vi "Write Sub Panel.vi"(8 "error in (no error)":errorcluster, 10 "Sub Panel":refnum<vi>, 11 "Window with subpanel in":refnum<class "Window with subpanel.lvclass">) -> (0 "error out":errorcluster, 3 "Window with subpanel out":refnum<class "Window with subpanel.lvclass">)   [LabVIEW 2020, in "Panel Form Tier Controllers.lvlib" / "Window with subpanel.lvclass"]
uses:
  Window with subpanel.lvclass
  Window with subpanel.lvclass/Window with subpanel.ctl
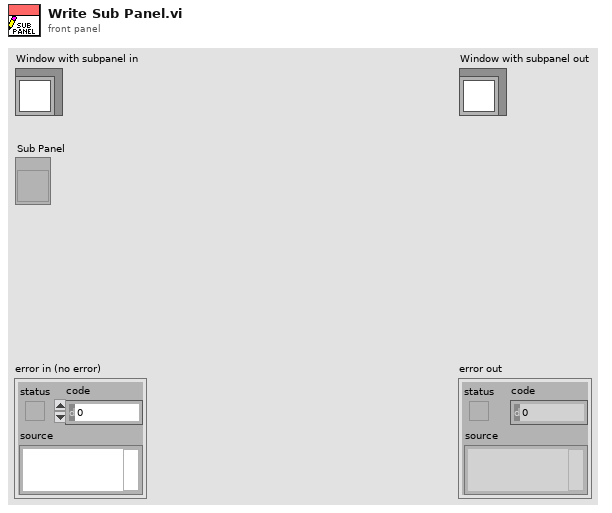
[diagram p1: front panel]
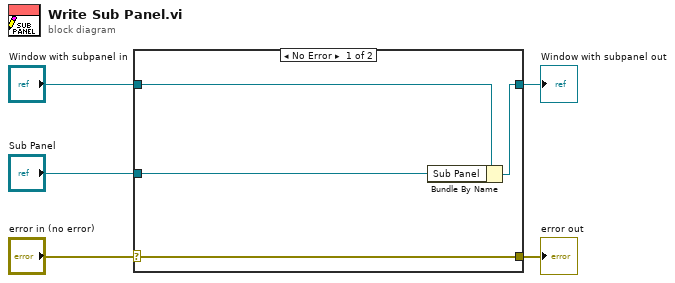
[diagram p0: block diagram]
diagram:
  n1 = case shown="No Error" "error in (no error)" {
    selector: "error in (no error)" -> [w9 w10]
    tunnel: [w9 w10] -> w4
    tunnel: [w7 w11] -> w2
    tunnel: "Window with subpanel in" -> [w8 w11]
    tunnel: "Sub Panel" -> [w6 _]
    frame No Error {
      n2 = Bundle By Name(cluster=w8, "Sub Panel"=w6) -> (w7:refnum<class "Window with subpanel.lvclass">)
    }
    frame Error {
    }
  }
  "error out" <- w4
  "Window with subpanel out" <- w2
